vi "pickAllyTeam.vi"(0 "object in":refnum<class "Ally.lvclass">, 2 "AllyRef":refnum<class "Robot.lvclass">[](array[class]), 3 "team":T1, 4 "allyTeamArray":T1[](array[typedef]), 5 "error in (no error)":errorcluster) -> (14 "object out":refnum<class "Ally.lvclass">, 16 "activeTeam":refnum<class "Robot.lvclass">[](array[class]), 19 "error out":errorcluster)   [LabVIEW 2023, in "Ally.lvclass"]
uses:
  Ally.lvclass
  STP_Parameters/AllyTeam.ctl
  Robot_class/Robot.lvclass
  Utilities_class/Utilities.lvclass
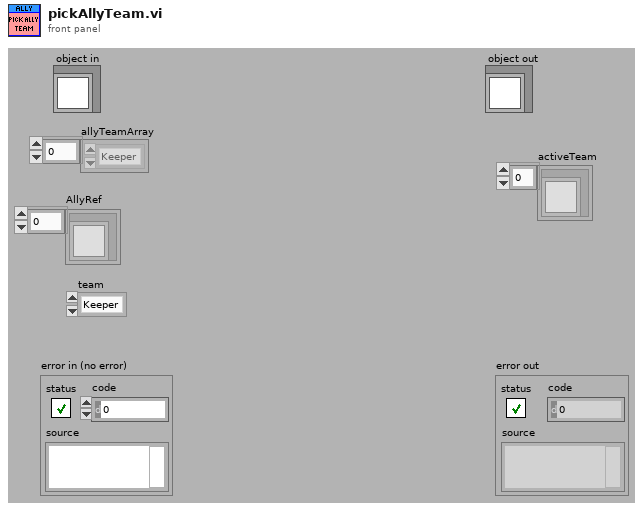
[diagram p1: front panel]
types:
  T1 = typedef "AllyTeam.ctl" = enum16{"Keeper", "Defender", "Attacker"}
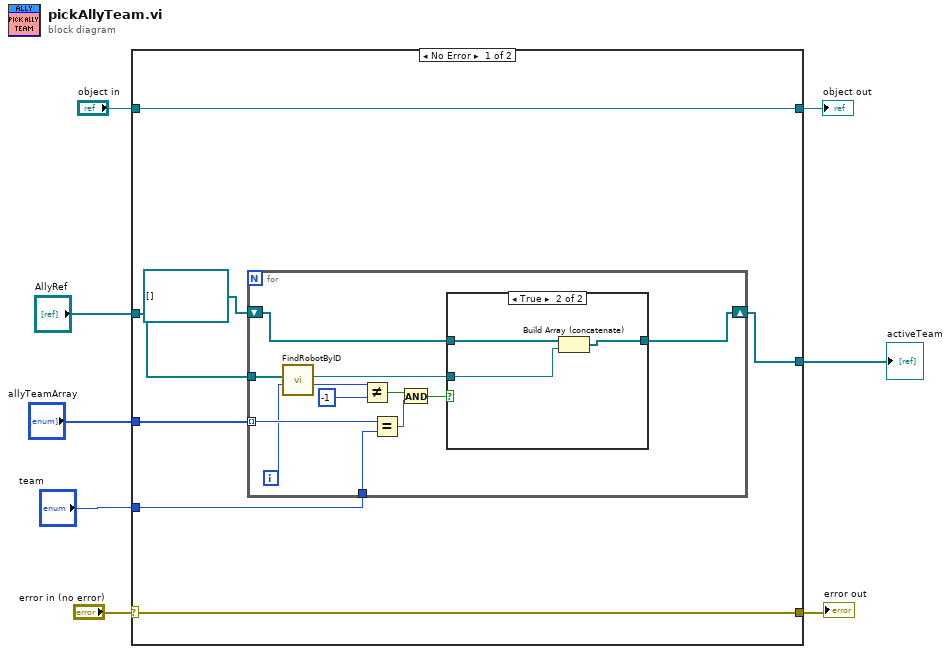
[diagram p0: block diagram]
diagram:
  n1 = case shown="No Error" "error in (no error)" {
    selector: "error in (no error)" -> [w15 w34]
    tunnel: [w15 w34] -> w7
    tunnel: [w14 w33] -> w5
    tunnel: "object in" -> [w14 w33]
    tunnel: "AllyRef" -> [w9 w32]
    tunnel: "allyTeamArray" -> [w12 _]
    tunnel: "team" -> [w11 _]
    tunnel: [w10 w32] -> w1
    frame No Error {
      n2 = for {
        tunnel: w12 -> [w27] mode=indexing
        shift-right: [w25] -> w10
        shift-left: refnum<class "Robot.lvclass">[] [] ("RobotRef") -> [w26]
        tunnel: w11 -> [w17]
        tunnel: w9 -> [w16]
        i -> [w22]
        n3 = call "FindRobotByID.vi"("id"=w22, "RobotRef"=w16) -> ("index"=w24:i32, "Robot"=w18:refnum<class "Robot.lvclass">)  [unwired: 6 in, 2 out]
        n4 = Not Equal?(x=w24, y=-1) -> (x != y?=w21:bool)
        n5 = Equal?(x=w27, y=w17) -> (x = y?=w19:bool)
        n6 = And(x=w21, y=w19) -> (x .and. y?=w20:bool)
        n7 = case shown="True" w20 {
          tunnel: w26 -> [w28 w31]
          tunnel: [w28 w30] -> w25
          tunnel: w18 -> [_ w29]
          frame False {
          }
          frame True {
            n8 = Build Array (concatenate)(w31, w29) -> (w30:refnum<class "Robot.lvclass">[])
          }
        }
      }
    }
    frame Error {
    }
  }
  "error out" <- w7
  "object out" <- w5
  "activeTeam" <- w1
